vi "VI Server_TREE_PopulateTreeItems_MultiSlot.vi"(4 "Item Names":string[][](array[string])=[["AI Test", "0", "AI Test", "AI Test", "-1.000", "", "1.000", "V"], ["fgggggggggggg", "1", "hggggggggg", "jjjjjjjjjjjjjjjjjj", "-1.000", "", "1.000", "V"], ["fgggggggggggg", "1", "hggggggggg", "jjjjjjjjjjjjjjjjjj", "-1.000", "", "1.000", "V"], ["fgggggggggggg", "1", "hggggggggg", "jjjjjjjjjjjjjjjjjj", "-1.000", "", "1.000", "V"], ["fgggggggggggg", "1", "hggggggggg", "jjjjjjjjjjjjjjjjjj", "-1.000", "", "1.000", "V"], ["fgggggggggggg", "1", "hggggggggg", "jjjjjjjjjjjjjjjjjj", "-1.000", "", "1.000", "V"], ["fgggggggggggg", "1", "hggggggggg", "jjjjjjjjjjjjjjjjjj", "-1.000", "", "1.000", "V"], ["fgggggggggggg", "1", "hggggggggg", "jjjjjjjjjjjjjjjjjj", "-1.000", "", "1.000", "V"], ["fgggggggggggg", "1", "hggggggggg", "jjjjjjjjjjjjjjjjjj", "-1.000", "", "1.000", "V"], ["fgggggggggggg", "1", "hggggggggg", "jjjjjjjjjjjjjjjjjj", "-1.000", "", "1.000", "V"], ["fgggggggggggg", "1", "hggggggggg", "jjjjjjjjjjjjjjjjjj", "-1.000", "", "1.000", "V"], ["Last Test Case", "1", "Description", "Conditions", "-1.000", "", "1.000", "V"]], 6 "Tree.RowHeaders":string[](array[string])=["1", "1.2", "1.3", "1.4", "1.5", "1.6", "1.9", "1.25", "2.2", "3.3", "3.6", "3.7"], 7 "Label":string="Test.Tree", 8 "error in":errorcluster, 9 "Tree.Ref":refnum<vi>, 11 "VI Server.RefsCluster":T1={"Labels"=["EXIT", "Test.Start", "Test.ABORT", "Test.Pause", "error in", "Login.Level", "Login.Name", "Help", "System.Message", "Instruments.Status", "Tab.Main", "Test.Tree", "Test.P/N", "Messages & Status", "Test.Progress", "Test.ElapsedTime", "Test.Repeat.RunOf", "Test.Repeat.NumberOfFailures", "SerialNumbers.Array", "Settings.P/N", "TestCase", "TestConfiguration", "TestCase.Description", "TestCase.Conditions", "TestCase.Parameter", "TestCaseConfiguration", "TestCase.TraceLimits", "TestCase.Function", "TestCase.Function.Argument1", "TestCase.Function.Argument2", "TestCase.Function.Argument3", "TestCase.Function.Argument3.DBL", "TestCase.LimitsIndex", "LimitsIndex.New", "Limit.Hi", "Limit.Lo", "Limit.Units", "Limits.SAVE", "Limits.Remove", "TestCase.Instrument.Data", "TestCase.InstrumentData.InRange", "TestCase.Execute.Selected", "TestCase.Execute.All", "TestCase.Execute.Pause", "TestCase.Execute.ABORT", "TestCase.Execute.Instruction", "TestCase.Add.Instruction", "TestCase.SAVE", "TestCase.Execution.StepTime", "TestCase.Update.Instruction", "Limit.Message", "TestCase.Execute.Pass/Fail", "Performance.Verification.Pass/Fail", "Performance.Verification.SAVE", "TestCase.Execute.Next", "TestConfiguration.RunAll", "TestConfiguration.Execute.Pass/Fail", "TestCaseExecution.StopOnFailure", "TestConfiguration.Run.Step", "TestCase.Add.Instruction.Pos", "TestCase.Execute.Steps", "TestCase.Execute.Step.Pause", "TestCase.ExecutionTime", "TestCase.StepDescription", "Limit.PicturePath", "TestCase.SAVE.Success", "TestCase.Function.Argument3.STR", "Fixture.SlotSelector", "Test.StartTime", "Test.EndTime", "TestCase.Instrument.Data.Str", "Graph1", "Graph2", "Image1", "Image2", "Image3", "Mem1", "Mem2", "Mem3", "Mem4", "Mem5", "Mem6", "Mem7", "Mem8", "Mem9", "Mem10", "Mem11", "Mem12", "Mem13", "Mem14", "Mem15", "Mem16", "Mem97", "Mem98", "Mem99", "Mem100", "Mem101", "Mem102", "Mem103", "Mem104", "Mem105", "Mem106", "Mem107", "Mem108", "Mem109", "Mem110", "Mem111", "Mem112", "Mem17", "Mem18", "Mem19", "Mem20", "Mem21", "Mem22", "Mem23", "Mem24", "Mem25", "Mem26", "Mem27", "Mem28", "Mem29", "Mem30", "Mem31", "Mem32", "Mem113", "Mem114", "Mem115", "Mem116", "Mem117", "Mem118", "Mem119", "Mem120", "Mem121", "Mem122", "Mem123", "Mem124", "Mem125", "Mem126", "Mem127", "Mem128", "Mem33", "Mem34", "Mem35", "Mem36", "Mem37", "Mem38", "Mem39", "Mem40", "Mem41", "Mem42", "Mem43", "Mem44", "Mem45", "Mem46", "Mem47", "Mem48", "Mem129", "Mem130", "Mem131", "Mem132", "Mem133", "Mem134", "Mem135", "Mem136", "Mem137", "Mem138", "Mem139", "Mem140", "Mem141", "Mem142", "Mem143", "Mem144", "Mem49", "Mem50", "Mem51", "Mem52", "Mem53", "Mem54", "Mem55", "Mem56", "Mem57", "Mem58", "Mem59", "Mem60", "Mem61", "Mem62", "Mem63", "Mem64", "Mem145", "Mem146", "Mem147", "Mem148", "Mem149", "Mem150", "Mem151", "Mem152", "Mem153", "Mem154", "Mem155", "Mem156", "Mem157", "Mem158", "Mem159", "Mem160", "Mem65", "Mem66", "Mem67", "Mem68", "Mem69", "Mem70", "Mem71", "Mem72", "Mem73", "Mem74", "Mem75", "Mem76", "Mem77", "Mem78", "Mem79", "Mem80", "Mem161", "Mem162", "Mem163", "Mem164", "Mem165", "Mem166", "Mem167", "Mem168", "Mem169", "Mem170", "Mem171", "Mem172", "Mem173", "Mem174", "Mem175", "Mem176", "Mem81", "Mem82", "Mem83", "Mem84", "Mem85", "Mem86", "Mem87", "Mem88", "Mem89", "Mem90", "Mem91", "Mem92", "Mem93", "Mem94", "Mem95", "Mem96", "Mem177", "Mem178", "Mem179", "Mem180", "Mem181", "Mem182", "Mem183", "Mem184", "Mem185", "Mem186", "Mem187", "Mem188", "Mem189", "Mem190", "Mem191", "Mem192", "Mem.RST", "Mem.Str.RST", "Mem.Str1", "Mem.Str2", "Mem.Str3", "Mem.Str4", "Mem.Str5", "Mem.Str6", "Mem.Str7", "Mem.Str1 8", "Mem.Str9", "Mem.Str10", "Mem.Str11", "Mem.Str12", "Mem.Str13", "Mem.Str14", "Mem.Str15", "Mem.Str16", "Mem.Str17", "Mem.Str18", "Mem.Str19", "Mem.Str20", "Mem.Str21", "Mem.Str22", "Mem.Str23", "Mem.Str24", "Mem.Str25", "Mem.Str26", "Mem.Str27", "Mem.Str28", "Mem.Str29", "Mem.Str30", "Mem.Str31", "Mem.Str32", "Mem.Str33", "Mem.Str34", "Mem.Str35", "Mem.Str36", "Mem.Str37", "Mem.Str38", "Mem.Str39", "Mem.Str40", "Mem.Str41", "Mem.Str42", "Mem.Str43", "Mem.Str44", "Mem.Str45", "Mem.Str46", "Mem.Str47", "Mem.Str48", "Mem.Str49", "Mem.Str50", "Mem.Str51", "Mem.Str52", "Mem.Str53", "Mem.Str54", "Mem.Str55", "Mem.Str56", "Mem.Str57", "Mem.Str58", "Mem.Str59", "Mem.Str60", "Mem.Str61", "Mem.Str62", "Mem.Str63", "Mem.Str64", "Mem.Str65", "Mem.Str66", "Mem.Str67", "Mem.Str68", "Mem.Str69", "Mem.Str70", "Mem.Str71", "Mem.Str72", "Mem.Str73", "Mem.Str74", "Mem.Str75", "Mem.Str76", "Mem.Str77", "Mem.Str78", "Mem.Str79", "Mem.Str80", "Mem.Str81", "Mem.Str82", "Mem.Str83", "Mem.Str84", "Mem.Str85", "Mem.Str86", "Mem.Str87", "Mem.Str88", "Mem.Str89", "Mem.Str90", "Mem.Str91", "Mem.Str92", "Mem.Str93", "Mem.Str94", "Mem.Str95", "Mem.Str96", "Mem.Str97", "Mem.Str98", "Mem.Str99", "Mem.Str100", "Mem.Str101", "Mem.Str102", "Mem.Str103", "Mem.Str104", "Mem.Str105", "Mem.Str106", "Mem.Str107", "Mem.Str108", "Mem.Str109", "Mem.Str110", "Mem.Str111", "Mem.Str112", "Mem.Str113", "Mem.Str114", "Mem.Str115", "Mem.Str116", "Mem.Str117", "Mem.Str118", "Mem.Str119", "Mem.Str120", "Mem.Str121", "Mem.Str122", "Mem.Str123", "Mem.Str124", "Mem.Str125", "Mem.Str126", "Mem.Str127", "Mem.Str128", "Mem.Str129", "Mem.Str130", "Mem.Str131", "Mem.Str132", "Mem.Str133", "Mem.Str134", "Mem.Str135", "Mem.Str136", "Mem.Str137", "Mem.Str138", "Mem.Str139", "Mem.Str140", "Mem.Str141", "Mem.Str142", "Mem.Str143", "Mem.Str144", "Mem.Str145", "Mem.Str146", "Mem.Str147", "Mem.Str148", "Mem.Str149", "Mem.Str150", "Mem.Str151", "Mem.Str152", "Mem.Str153", "Mem.Str154", "Mem.Str155", "Mem.Str156", "Mem.Str157", "Mem.Str158", "Mem.Str159", "Mem.Str160", "Mem.Str161", "Mem.Str162", "Mem.Str163", "Mem.Str164", "Mem.Str165", "Mem.Str166", "Mem.Str167", "Mem.Str168", "Mem.Str169", "Mem.Str170", "Mem.Str171", "Mem.Str172", "Mem.Str173", "Mem.Str174", "Mem.Str175 2", "Mem.Str175", "Mem.Str177", "Mem.Str178", "Mem.Str179", "Mem.Str180", "Mem.Str181", "Mem.Str182", "Mem.Str183", "Mem.Str184", "Mem.Str185", "Mem.Str186", "Mem.Str187", "Mem.Str188", "Mem.Str189", "Mem.Str190", "Mem.Str191", "Mem.Str192", "Report.PDF.File", "Report.PDF.File.Content", "Report.PDF.File.Read", "Report.PDF.File.Content.Clear", "error out", "UDP.IP.Address", "UDP.LocalPort", "UDP.Port.BC", "UDP.Port.RT", "UDP.Test.String", "UDP.Responce.String", "UDP.Responce.String.Monitor", "UDP.Test.String.Send", "Instr.Responce.Timeout", "UDP.Sent.String", "Performance.Verification.Enable", "UDP.Responce.Array", "UDP.Write.Array", "TestCase.Diagnostics.ABORT", "TestCase.Diagnostics.Pause", "TestCase.Diagnostics.Next", "TestCase.Diagnostics.Instruction", "InstrumentLoad.Disable", "TestTree.CollapseItems", "Test.Repeat.NumberOf", "Test.Results.LogFile.Folder", "Report.Test", "Test.Report.Skip", "Report.MS_Word.Path", "Setup.AdobeAcrobat.Path", "Test.Instruments.FP", "UDP.Responce.Array.EmptyAtStart", "UDP.Test.String2", "UDP.Test.String2.Send", "CodeTest.Start", "Help.Enable", "Fixture.Slot1", "Fixture.Slot2", "Fixture.Slot3", "Fixture.Slot4", "Fixture.Slot5", "Fixture.Slot6", "Fixture.Slot7", "Fixture.Slot8", "Users", "Users.Load", "Users.Name", "Users.Level", "User.AddNew", "User.Remove", "User.SAVE", "User.Password"], "Refs"=[refnum, refnum, refnum, refnum, refnum, refnum, refnum, refnum, refnum, refnum, refnum, refnum, refnum, refnum, refnum, refnum, refnum, refnum, refnum, refnum, refnum, refnum, refnum, refnum, refnum, refnum, refnum, refnum, refnum, refnum, refnum, refnum, refnum, refnum, refnum, refnum, refnum, refnum, refnum, refnum, refnum, refnum, refnum, refnum, refnum, refnum, refnum, refnum, refnum, refnum, refnum, refnum, refnum, refnum, refnum, refnum, refnum, refnum, refnum, refnum, refnum, refnum, refnum, refnum, refnum, refnum, refnum, refnum, refnum, refnum, refnum, refnum, refnum, refnum, refnum, refnum, refnum, refnum, refnum, refnum, refnum, refnum, refnum, refnum, refnum, refnum, refnum, refnum, refnum, refnum, refnum, refnum, refnum, refnum, refnum, refnum, refnum, refnum, refnum, refnum, refnum, refnum, refnum, refnum, refnum, refnum, refnum, refnum, refnum, refnum, refnum, refnum, refnum, refnum, refnum, refnum, refnum, refnum, refnum, refnum, refnum, refnum, refnum, refnum, refnum, refnum, refnum, refnum, refnum, refnum, refnum, refnum, refnum, refnum, refnum, refnum, refnum, refnum, refnum, refnum, refnum, refnum, refnum, refnum, refnum, refnum, refnum, refnum, refnum, refnum, refnum, refnum, refnum, refnum, refnum, refnum, refnum, refnum, refnum, refnum, refnum, refnum, refnum, refnum, refnum, refnum, refnum, refnum, refnum, refnum, refnum, refnum, refnum, refnum, refnum, refnum, refnum, refnum, refnum, refnum, refnum, refnum, refnum, refnum, refnum, refnum, refnum, refnum, refnum, refnum, refnum, refnum, refnum, refnum, refnum, refnum, refnum, refnum, refnum, refnum, refnum, refnum, refnum, refnum, refnum, refnum, refnum, refnum, refnum, refnum, refnum, refnum, refnum, refnum, refnum, refnum, refnum, refnum, refnum, refnum, refnum, refnum, refnum, refnum, refnum, refnum, refnum, refnum, refnum, refnum, refnum, refnum, refnum, refnum, refnum, refnum, refnum, refnum, refnum, refnum, refnum, refnum, refnum, refnum, refnum, refnum, refnum, refnum, refnum, refnum, refnum, refnum, refnum, refnum, refnum, refnum, refnum, refnum, refnum, refnum, refnum, refnum, refnum, refnum, refnum, refnum, refnum, refnum, refnum, refnum, refnum, refnum, refnum, refnum, refnum, refnum, refnum, refnum, refnum, refnum, refnum, refnum, refnum, refnum, refnum, refnum, refnum, refnum, refnum, refnum, refnum, refnum, refnum, refnum, refnum, refnum, refnum, refnum, refnum, refnum, refnum, refnum, refnum, refnum, refnum, refnum, refnum, refnum, refnum, refnum, refnum, refnum, refnum, refnum, refnum, refnum, refnum, refnum, refnum, refnum, refnum, refnum, refnum, refnum, refnum, refnum, refnum, refnum, refnum, refnum, refnum, refnum, refnum, refnum, refnum, refnum, refnum, refnum, refnum, refnum, refnum, refnum, refnum, refnum, refnum, refnum, refnum, refnum, refnum, refnum, refnum, refnum, refnum, refnum, refnum, refnum, refnum, refnum, refnum, refnum, refnum, refnum, refnum, refnum, refnum, refnum, refnum, refnum, refnum, refnum, refnum, refnum, refnum, refnum, refnum, refnum, refnum, refnum, refnum, refnum, refnum, refnum, refnum, refnum, refnum, refnum, refnum, refnum, refnum, refnum, refnum, refnum, refnum, refnum, refnum, refnum, refnum, refnum, refnum, refnum, refnum, refnum, refnum, refnum, refnum, refnum, refnum, refnum, refnum, refnum, refnum, refnum, refnum, refnum, refnum, refnum, refnum, refnum, refnum, refnum, refnum, refnum, refnum, refnum, refnum, refnum, refnum, refnum, refnum, refnum, refnum, refnum, refnum, refnum, refnum, refnum, refnum, refnum, refnum, refnum, refnum, refnum, refnum, refnum, refnum, refnum, refnum, refnum, refnum, refnum, refnum, refnum, refnum, refnum, refnum, refnum, refnum, refnum, refnum, refnum, refnum, refnum, refnum, refnum, refnum, refnum, refnum, refnum, refnum, refnum, refnum, refnum, refnum, refnum, refnum, refnum, refnum, refnum, refnum, refnum, refnum, refnum, refnum, refnum, refnum, refnum, refnum, refnum, refnum, refnum, refnum, refnum, refnum, refnum, refnum, refnum, refnum, refnum, refnum, refnum, refnum, refnum, refnum, refnum, refnum, refnum, refnum, refnum, refnum, refnum, refnum, refnum, refnum, refnum], "VI Ref"=refnum}) -> (0 "error out":errorcluster, 1 "Tree.Ref.DUP":refnum<vi>, 3 "VI Server.RefsCluster.DUP":T1={"Labels"=["EXIT", "Test.Start", "Test.ABORT", "Test.Pause", "error in", "Login.Level", "Login.Name", "Help", "System.Message", "Instruments.Status", "Tab.Main", "Test.Tree", "Test.P/N", "Messages & Status", "Test.Progress", "Test.ElapsedTime", "Test.Repeat.RunOf", "Test.Repeat.NumberOfFailures", "SerialNumbers.Array", "Settings.P/N", "TestCase", "TestConfiguration", "TestCase.Description", "TestCase.Conditions", "TestCase.Parameter", "TestCaseConfiguration", "TestCase.TraceLimits", "TestCase.Function", "TestCase.Function.Argument1", "TestCase.Function.Argument2", "TestCase.Function.Argument3", "TestCase.Function.Argument3.DBL", "TestCase.LimitsIndex", "LimitsIndex.New", "Limit.Hi", "Limit.Lo", "Limit.Units", "Limits.SAVE", "Limits.Remove", "TestCase.Instrument.Data", "TestCase.InstrumentData.InRange", "TestCase.Execute.Selected", "TestCase.Execute.All", "TestCase.Execute.Pause", "TestCase.Execute.ABORT", "TestCase.Execute.Instruction", "TestCase.Add.Instruction", "TestCase.SAVE", "TestCase.Execution.StepTime", "TestCase.Update.Instruction", "Limit.Message", "TestCase.Execute.Pass/Fail", "Performance.Verification.Pass/Fail", "Performance.Verification.SAVE", "TestCase.Execute.Next", "TestConfiguration.RunAll", "TestConfiguration.Execute.Pass/Fail", "TestCaseExecution.StopOnFailure", "TestConfiguration.Run.Step", "TestCase.Add.Instruction.Pos", "TestCase.Execute.Steps", "TestCase.Execute.Step.Pause", "TestCase.ExecutionTime", "TestCase.StepDescription", "Limit.PicturePath", "TestCase.SAVE.Success", "TestCase.Function.Argument3.STR", "Fixture.SlotSelector", "Test.StartTime", "Test.EndTime", "TestCase.Instrument.Data.Str", "Graph1", "Graph2", "Image1", "Image2", "Image3", "Mem1", "Mem2", "Mem3", "Mem4", "Mem5", "Mem6", "Mem7", "Mem8", "Mem9", "Mem10", "Mem11", "Mem12", "Mem13", "Mem14", "Mem15", "Mem16", "Mem97", "Mem98", "Mem99", "Mem100", "Mem101", "Mem102", "Mem103", "Mem104", "Mem105", "Mem106", "Mem107", "Mem108", "Mem109", "Mem110", "Mem111", "Mem112", "Mem17", "Mem18", "Mem19", "Mem20", "Mem21", "Mem22", "Mem23", "Mem24", "Mem25", "Mem26", "Mem27", "Mem28", "Mem29", "Mem30", "Mem31", "Mem32", "Mem113", "Mem114", "Mem115", "Mem116", "Mem117", "Mem118", "Mem119", "Mem120", "Mem121", "Mem122", "Mem123", "Mem124", "Mem125", "Mem126", "Mem127", "Mem128", "Mem33", "Mem34", "Mem35", "Mem36", "Mem37", "Mem38", "Mem39", "Mem40", "Mem41", "Mem42", "Mem43", "Mem44", "Mem45", "Mem46", "Mem47", "Mem48", "Mem129", "Mem130", "Mem131", "Mem132", "Mem133", "Mem134", "Mem135", "Mem136", "Mem137", "Mem138", "Mem139", "Mem140", "Mem141", "Mem142", "Mem143", "Mem144", "Mem49", "Mem50", "Mem51", "Mem52", "Mem53", "Mem54", "Mem55", "Mem56", "Mem57", "Mem58", "Mem59", "Mem60", "Mem61", "Mem62", "Mem63", "Mem64", "Mem145", "Mem146", "Mem147", "Mem148", "Mem149", "Mem150", "Mem151", "Mem152", "Mem153", "Mem154", "Mem155", "Mem156", "Mem157", "Mem158", "Mem159", "Mem160", "Mem65", "Mem66", "Mem67", "Mem68", "Mem69", "Mem70", "Mem71", "Mem72", "Mem73", "Mem74", "Mem75", "Mem76", "Mem77", "Mem78", "Mem79", "Mem80", "Mem161", "Mem162", "Mem163", "Mem164", "Mem165", "Mem166", "Mem167", "Mem168", "Mem169", "Mem170", "Mem171", "Mem172", "Mem173", "Mem174", "Mem175", "Mem176", "Mem81", "Mem82", "Mem83", "Mem84", "Mem85", "Mem86", "Mem87", "Mem88", "Mem89", "Mem90", "Mem91", "Mem92", "Mem93", "Mem94", "Mem95", "Mem96", "Mem177", "Mem178", "Mem179", "Mem180", "Mem181", "Mem182", "Mem183", "Mem184", "Mem185", "Mem186", "Mem187", "Mem188", "Mem189", "Mem190", "Mem191", "Mem192", "Mem.RST", "Mem.Str.RST", "Mem.Str1", "Mem.Str2", "Mem.Str3", "Mem.Str4", "Mem.Str5", "Mem.Str6", "Mem.Str7", "Mem.Str1 8", "Mem.Str9", "Mem.Str10", "Mem.Str11", "Mem.Str12", "Mem.Str13", "Mem.Str14", "Mem.Str15", "Mem.Str16", "Mem.Str17", "Mem.Str18", "Mem.Str19", "Mem.Str20", "Mem.Str21", "Mem.Str22", "Mem.Str23", "Mem.Str24", "Mem.Str25", "Mem.Str26", "Mem.Str27", "Mem.Str28", "Mem.Str29", "Mem.Str30", "Mem.Str31", "Mem.Str32", "Mem.Str33", "Mem.Str34", "Mem.Str35", "Mem.Str36", "Mem.Str37", "Mem.Str38", "Mem.Str39", "Mem.Str40", "Mem.Str41", "Mem.Str42", "Mem.Str43", "Mem.Str44", "Mem.Str45", "Mem.Str46", "Mem.Str47", "Mem.Str48", "Mem.Str49", "Mem.Str50", "Mem.Str51", "Mem.Str52", "Mem.Str53", "Mem.Str54", "Mem.Str55", "Mem.Str56", "Mem.Str57", "Mem.Str58", "Mem.Str59", "Mem.Str60", "Mem.Str61", "Mem.Str62", "Mem.Str63", "Mem.Str64", "Mem.Str65", "Mem.Str66", "Mem.Str67", "Mem.Str68", "Mem.Str69", "Mem.Str70", "Mem.Str71", "Mem.Str72", "Mem.Str73", "Mem.Str74", "Mem.Str75", "Mem.Str76", "Mem.Str77", "Mem.Str78", "Mem.Str79", "Mem.Str80", "Mem.Str81", "Mem.Str82", "Mem.Str83", "Mem.Str84", "Mem.Str85", "Mem.Str86", "Mem.Str87", "Mem.Str88", "Mem.Str89", "Mem.Str90", "Mem.Str91", "Mem.Str92", "Mem.Str93", "Mem.Str94", "Mem.Str95", "Mem.Str96", "Mem.Str97", "Mem.Str98", "Mem.Str99", "Mem.Str100", "Mem.Str101", "Mem.Str102", "Mem.Str103", "Mem.Str104", "Mem.Str105", "Mem.Str106", "Mem.Str107", "Mem.Str108", "Mem.Str109", "Mem.Str110", "Mem.Str111", "Mem.Str112", "Mem.Str113", "Mem.Str114", "Mem.Str115", "Mem.Str116", "Mem.Str117", "Mem.Str118", "Mem.Str119", "Mem.Str120", "Mem.Str121", "Mem.Str122", "Mem.Str123", "Mem.Str124", "Mem.Str125", "Mem.Str126", "Mem.Str127", "Mem.Str128", "Mem.Str129", "Mem.Str130", "Mem.Str131", "Mem.Str132", "Mem.Str133", "Mem.Str134", "Mem.Str135", "Mem.Str136", "Mem.Str137", "Mem.Str138", "Mem.Str139", "Mem.Str140", "Mem.Str141", "Mem.Str142", "Mem.Str143", "Mem.Str144", "Mem.Str145", "Mem.Str146", "Mem.Str147", "Mem.Str148", "Mem.Str149", "Mem.Str150", "Mem.Str151", "Mem.Str152", "Mem.Str153", "Mem.Str154", "Mem.Str155", "Mem.Str156", "Mem.Str157", "Mem.Str158", "Mem.Str159", "Mem.Str160", "Mem.Str161", "Mem.Str162", "Mem.Str163", "Mem.Str164", "Mem.Str165", "Mem.Str166", "Mem.Str167", "Mem.Str168", "Mem.Str169", "Mem.Str170", "Mem.Str171", "Mem.Str172", "Mem.Str173", "Mem.Str174", "Mem.Str175 2", "Mem.Str175", "Mem.Str177", "Mem.Str178", "Mem.Str179", "Mem.Str180", "Mem.Str181", "Mem.Str182", "Mem.Str183", "Mem.Str184", "Mem.Str185", "Mem.Str186", "Mem.Str187", "Mem.Str188", "Mem.Str189", "Mem.Str190", "Mem.Str191", "Mem.Str192", "Report.PDF.File", "Report.PDF.File.Content", "Report.PDF.File.Read", "Report.PDF.File.Content.Clear", "error out", "UDP.IP.Address", "UDP.LocalPort", "UDP.Port.BC", "UDP.Port.RT", "UDP.Test.String", "UDP.Responce.String", "UDP.Responce.String.Monitor", "UDP.Test.String.Send", "Instr.Responce.Timeout", "UDP.Sent.String", "Performance.Verification.Enable", "UDP.Responce.Array", "UDP.Write.Array", "TestCase.Diagnostics.ABORT", "TestCase.Diagnostics.Pause", "TestCase.Diagnostics.Next", "TestCase.Diagnostics.Instruction", "InstrumentLoad.Disable", "TestTree.CollapseItems", "Test.Repeat.NumberOf", "Test.Results.LogFile.Folder", "Report.Test", "Test.Report.Skip", "Report.MS_Word.Path", "Setup.AdobeAcrobat.Path", "Test.Instruments.FP", "UDP.Responce.Array.EmptyAtStart", "UDP.Test.String2", "UDP.Test.String2.Send", "CodeTest.Start", "Help.Enable", "Fixture.Slot1", "Fixture.Slot2", "Fixture.Slot3", "Fixture.Slot4", "Fixture.Slot5", "Fixture.Slot6", "Fixture.Slot7", "Fixture.Slot8", "Users", "Users.Load", "Users.Name", "Users.Level", "User.AddNew", "User.Remove", "User.SAVE", "User.Password"], "Refs"=[refnum, refnum, refnum, refnum, refnum, refnum, refnum, refnum, refnum, refnum, refnum, refnum, refnum, refnum, refnum, refnum, refnum, refnum, refnum, refnum, refnum, refnum, refnum, refnum, refnum, refnum, refnum, refnum, refnum, refnum, refnum, refnum, refnum, refnum, refnum, refnum, refnum, refnum, refnum, refnum, refnum, refnum, refnum, refnum, refnum, refnum, refnum, refnum, refnum, refnum, refnum, refnum, refnum, refnum, refnum, refnum, refnum, refnum, refnum, refnum, refnum, refnum, refnum, refnum, refnum, refnum, refnum, refnum, refnum, refnum, refnum, refnum, refnum, refnum, refnum, refnum, refnum, refnum, refnum, refnum, refnum, refnum, refnum, refnum, refnum, refnum, refnum, refnum, refnum, refnum, refnum, refnum, refnum, refnum, refnum, refnum, refnum, refnum, refnum, refnum, refnum, refnum, refnum, refnum, refnum, refnum, refnum, refnum, refnum, refnum, refnum, refnum, refnum, refnum, refnum, refnum, refnum, refnum, refnum, refnum, refnum, refnum, refnum, refnum, refnum, refnum, refnum, refnum, refnum, refnum, refnum, refnum, refnum, refnum, refnum, refnum, refnum, refnum, refnum, refnum, refnum, refnum, refnum, refnum, refnum, refnum, refnum, refnum, refnum, refnum, refnum, refnum, refnum, refnum, refnum, refnum, refnum, refnum, refnum, refnum, refnum, refnum, refnum, refnum, refnum, refnum, refnum, refnum, refnum, refnum, refnum, refnum, refnum, refnum, refnum, refnum, refnum, refnum, refnum, refnum, refnum, refnum, refnum, refnum, refnum, refnum, refnum, refnum, refnum, refnum, refnum, refnum, refnum, refnum, refnum, refnum, refnum, refnum, refnum, refnum, refnum, refnum, refnum, refnum, refnum, refnum, refnum, refnum, refnum, refnum, refnum, refnum, refnum, refnum, refnum, refnum, refnum, refnum, refnum, refnum, refnum, refnum, refnum, refnum, refnum, refnum, refnum, refnum, refnum, refnum, refnum, refnum, refnum, refnum, refnum, refnum, refnum, refnum, refnum, refnum, refnum, refnum, refnum, refnum, refnum, refnum, refnum, refnum, refnum, refnum, refnum, refnum, refnum, refnum, refnum, refnum, refnum, refnum, refnum, refnum, refnum, refnum, refnum, refnum, refnum, refnum, refnum, refnum, refnum, refnum, refnum, refnum, refnum, refnum, refnum, refnum, refnum, refnum, refnum, refnum, refnum, refnum, refnum, refnum, refnum, refnum, refnum, refnum, refnum, refnum, refnum, refnum, refnum, refnum, refnum, refnum, refnum, refnum, refnum, refnum, refnum, refnum, refnum, refnum, refnum, refnum, refnum, refnum, refnum, refnum, refnum, refnum, refnum, refnum, refnum, refnum, refnum, refnum, refnum, refnum, refnum, refnum, refnum, refnum, refnum, refnum, refnum, refnum, refnum, refnum, refnum, refnum, refnum, refnum, refnum, refnum, refnum, refnum, refnum, refnum, refnum, refnum, refnum, refnum, refnum, refnum, refnum, refnum, refnum, refnum, refnum, refnum, refnum, refnum, refnum, refnum, refnum, refnum, refnum, refnum, refnum, refnum, refnum, refnum, refnum, refnum, refnum, refnum, refnum, refnum, refnum, refnum, refnum, refnum, refnum, refnum, refnum, refnum, refnum, refnum, refnum, refnum, refnum, refnum, refnum, refnum, refnum, refnum, refnum, refnum, refnum, refnum, refnum, refnum, refnum, refnum, refnum, refnum, refnum, refnum, refnum, refnum, refnum, refnum, refnum, refnum, refnum, refnum, refnum, refnum, refnum, refnum, refnum, refnum, refnum, refnum, refnum, refnum, refnum, refnum, refnum, refnum, refnum, refnum, refnum, refnum, refnum, refnum, refnum, refnum, refnum, refnum, refnum, refnum, refnum, refnum, refnum, refnum, refnum, refnum, refnum, refnum, refnum, refnum, refnum, refnum, refnum, refnum, refnum, refnum, refnum, refnum, refnum, refnum, refnum, refnum, refnum, refnum, refnum, refnum, refnum, refnum, refnum, refnum, refnum, refnum, refnum, refnum, refnum, refnum, refnum, refnum, refnum, refnum, refnum, refnum, refnum, refnum, refnum, refnum, refnum, refnum, refnum, refnum, refnum, refnum, refnum, refnum, refnum, refnum, refnum, refnum, refnum, refnum, refnum, refnum, refnum, refnum, refnum, refnum, refnum, refnum, refnum, refnum, refnum, refnum, refnum, refnum, refnum, refnum, refnum, refnum, refnum, refnum], "VI Ref"=refnum})   [LabVIEW 2020]
uses:
  VI Server_TypeDefs/VI Server_RefsCluster.ctl
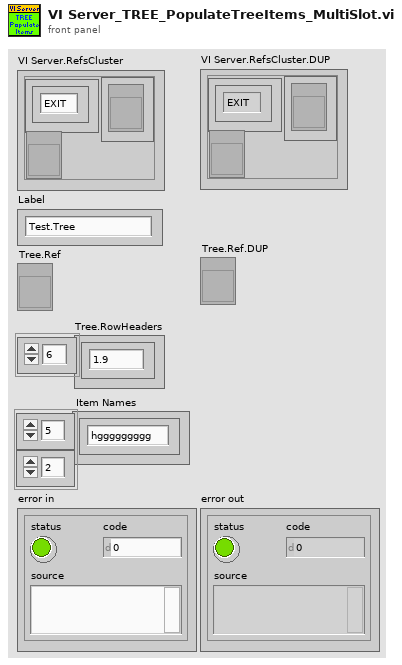
[diagram p1: front panel]
types:
  T1 = typedef "VI Server_RefsCluster.ctl" = cluster{"Labels":string[], "Refs":refnum<vi>[], "VI Ref":refnum<vi>}
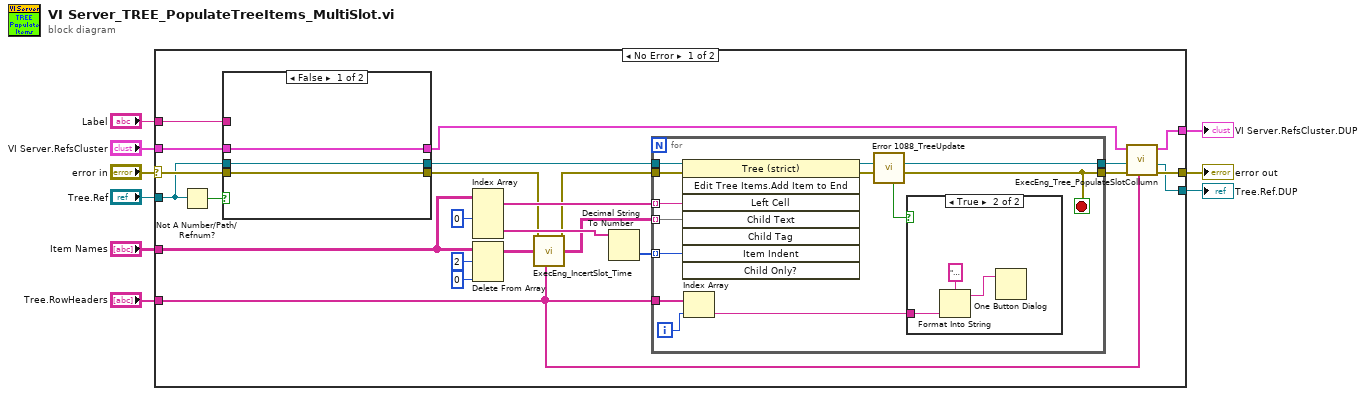
[diagram p0: block diagram]
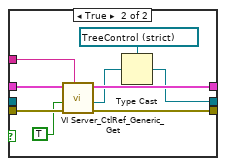
[diagram p3: hidden frame]
diagram:
  n1 = case shown="No Error" "error in" {
    selector: "error in" -> [w33 w62]
    tunnel: [w16 w62] -> w8
    tunnel: "VI Server.RefsCluster" -> [w32 w61]
    tunnel: [w14 w61] -> w7
    tunnel: "Label" -> [w22 _]
    tunnel: [w11 _] -> w3
    tunnel: "Tree.Ref" -> [w30 _]
    tunnel: "Item Names" -> [w21 _]
    tunnel: "Tree.RowHeaders" -> [w10 _]
    frame No Error {
      n2 = Not A Number/Path/Refnum?(number/path/refnum=w30) -> (NaN/Path/Refnum?=w31:bool)
      n3 = case shown="False" w31 {
        tunnel: w33 -> [w51 w60]
        tunnel: w32 -> [w50 w59]
        tunnel: [w50 w58] -> w13
        tunnel: w22 -> [_ w57]
        tunnel: [w51 w55] -> w18
        tunnel: w30 -> [w49 _]
        tunnel: [w49 w54] -> w23
        frame False {
        }
        frame True {
          n4 = call "VI Server_CtlRef_Generic_Get.vi"("Control.Label"=w57, "error in"=w60, "SingleInstance"=TRUE, "VI Server.RefsCluster"=w59) -> ("error out"=w55:errorcluster, "Control.Ref.Generic"=w56:refnum<vi>, "VI Server.RefsCluster.DUP"=w58:T1)  [unwired: 5 in]
          n5 = Type Cast(type=refnum<vi> refnum ("Test.Tree"), x=w56) -> (*(type *) &x=w54:refnum<vi>)
        }
      }
      n6 = Index Array(array=w21, index (col) #1=0 ("disabled index (col)")) -> (element #1=w28:string[], element #2=w27:string[])  [unwired: 3 in]
      n7 = Delete From Array(array=w21, length=2, index (col)=0 ("disabled index (col)")) -> (array with subset deleted=w20:string[][])  [unwired: 1 in, 1 out]
      n8 = call "ExecEng_IncertSlot_Time.vi"("error in"=w18, "Child.Text.In"=w20, "Tree.RowHeaders/TestCases"=w10) -> ("error out"=w17:errorcluster, "Child.Text.Out"=w19:string[][])  [unwired: 3 in]
      n9 = Decimal String To Number(string=w27) -> (number=w26:i32[])  [unwired: 2 in, 1 out]
      n10 = for {
        tunnel: w28 -> [w44] mode=indexing
        tunnel: w26 -> [w43] mode=indexing
        tunnel: w19 -> [w42] mode=indexing
        tunnel: [w41] -> w12
        tunnel: w17 -> [w45]
        tunnel: [w36] -> w15
        tunnel: w23 -> [w40]
        tunnel: w10 -> [w38]
        i -> [w39]
        stop <- w36 stop-if-true
        # "Populate the tree items"
        n11 = invoke on="Invoke Node" class="Tree (strict)" method="Edit Tree Items.Add Item to End"(reference=w40, error in=w45, "Left Cell"=w44, "Child Text"=w42, "Item Indent"=w43) -> (reference out=w41:refnum<vi>, error out=w37:errorcluster)  [unwired: 3 in, 6 out]
        n12 = Index Array(array=w38, index=w39) -> (element=w34:string)
        n13 = call "Error 1088_TreeUpdate.vi"("error in"=w37) -> ("error out"=w36:errorcluster, "Error.1088"=w35:bool)  [unwired: 9 in]
        n14 = case shown="True" w35 {
          tunnel: w34 -> [_ w48]
          frame False {
          }
          frame True {
            n15 = Format Into String(format string="Error loading Teast Case #%s.\nPossible Reason:\nThere is no parent item for this test case.\nAs an example, if the test case number is 2.1.1, there MUST be\nthe test case/item with number of 2.1", w48) -> (resulting string=w46:string)  [unwired: 2 in, 1 out]
            n16 = One Button Dialog(message=w46) -> ()  [unwired: 1 in, 1 out]
          }
        }
      }
      n17 = call "ExecEng_Tree_PopulateSlotCollumn.vi"("Tree.RowHeaders"=w10, "error in (no error)"=w15, "TreeControl.Ref"=w12, "VI Server.RefsCluster"=w13) -> ("error out"=w16:errorcluster, "TreeControl.Ref.DUP"=w11:refnum<vi>, "VI Server.RefsCluster.DUP"=w14:T1)  [unwired: 5 in]
    }
    frame Error {
    }
  }
  "error out" <- w8
  "Tree.Ref.DUP" <- w3
  "VI Server.RefsCluster.DUP" <- w7
